vi "configure.vi"(8 "error in (no error)":errorcluster, 9 "Value":i32, 10 "ILC":refnum<class "ILC.lvclass">, 11 "ConfigureILCSSRStrategy in":refnum<class "ConfigureILCDCADAC1Strategy.lvclass">) -> (0 "error out":errorcluster, 2 "ILC 2":refnum<class "ILC.lvclass">, 3 "ConfigureILCSSRStrategy out":refnum<class "ConfigureILCDCADAC1Strategy.lvclass">)   [LabVIEW 2016, in "ConfigureILCDCADAC1Strategy.lvclass"]
uses:
  ConfigureILCDCADAC1Strategy.lvclass
  Common_ILC/ILC/ILC.lvclass
  Common_ILC/ILC/ILC.lvclass/ILC.ctl
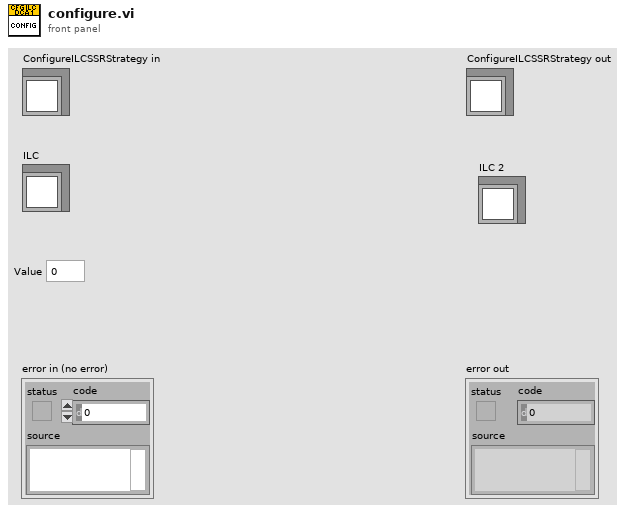
[diagram p1: front panel]
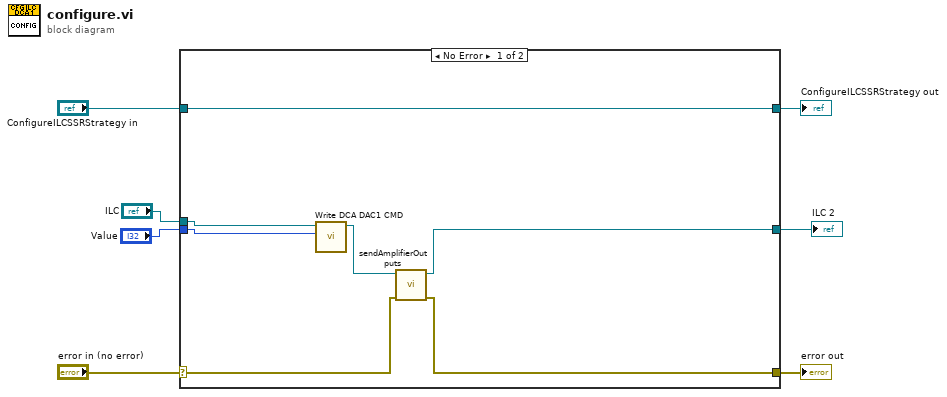
[diagram p0: block diagram]
diagram:
  n1 = case shown="No Error" "error in (no error)" {
    selector: "error in (no error)" -> [w10 w17]
    tunnel: [w9 w17] -> w6
    tunnel: [w14 w16] -> w4
    tunnel: "ConfigureILCSSRStrategy in" -> [w14 w16]
    tunnel: "ILC" -> [w13 w15]
    tunnel: "Value" -> [w12 _]
    tunnel: [w8 w15] -> w1
    frame No Error {
      n2 = call "Write DCA DAC1 CMD.vi"("DCA DAC1 CMD"=w12, "ILC in"=w13) -> ("ILC out"=w11:refnum<class "ILC.lvclass">)  [unwired: 9 in]
      n3 = call "sendAmplifierOutputs.vi"("error in (no error)"=w10, "ILC in"=w11) -> ("error out"=w9:errorcluster, "ILC out"=w8:refnum<class "ILC.lvclass">)  [unwired: 8 in]
    }
    frame Error {
    }
  }
  "error out" <- w6
  "ConfigureILCSSRStrategy out" <- w4
  "ILC 2" <- w1
